vi "Enable Disable Key Down Events.vi"(8 "error in (no error)":errorcluster, 10 "Enable?":bool, 11 "UI in":refnum<class "UI.lvclass">) -> (0 "error out":errorcluster)   [LabVIEW 2020, in "AR Example.lvlib" / "UI.lvclass"]
uses:
  UI.lvclass
  UI.lvclass/UI.ctl
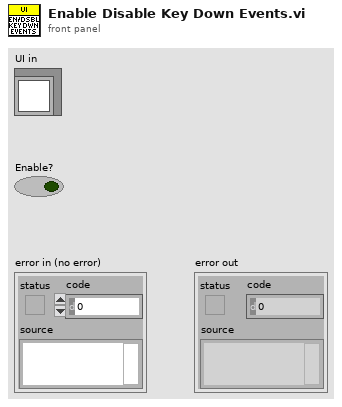
[diagram p1: front panel]
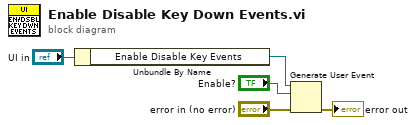
[diagram p0: block diagram]
diagram:
  n1 = Unbundle By Name("UI in") -> ("Enable Disable Key Events"=w4:refnum<user-event>)
  n2 = Generate User Event(user event=w4, event data cluster="Enable?", error in="error in (no error)") -> (error out=→"error out":errorcluster)  [unwired: 1 in, 1 out]
